vi "Untitled 1.vi"(9 "signal 3":waveform(dbl), 10 "signal 2":waveform(dbl), 11 "signal 1":waveform(dbl)) -> ()   [LabVIEW 2012]
panel:
  out "signal 3":dbl[](array[numeric])
  out "signal 2":dbl[](array[numeric])
  out "t":dbl[](array[numeric])
  out "signal 1":dbl[](array[numeric])
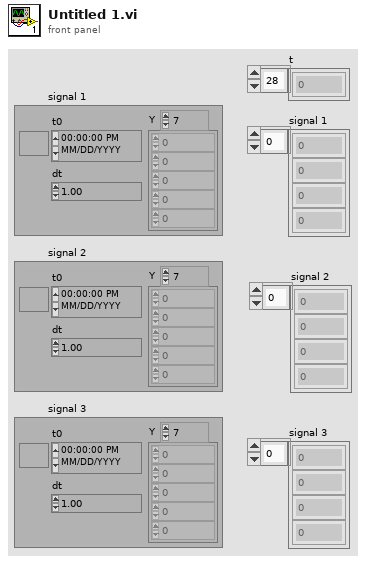
[diagram p1: front panel]
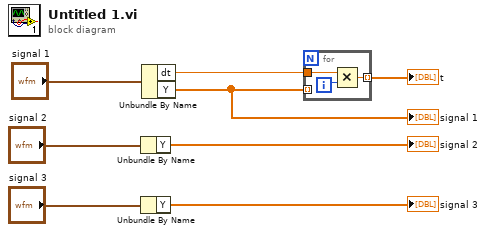
[diagram p0: block diagram]
diagram:
  n1 = Unbundle By Name("signal 2") -> ("Y"=→"signal 2":dbl[])
  n2 = Unbundle By Name("signal 3") -> ("Y"=→"signal 3":dbl[])
  n3 = Unbundle By Name("signal 1") -> ("dt"=w7:dbl, "Y"=w5:dbl[])
  "signal 1" <- w5
  n4 = for {
    tunnel: w7 -> [w11]
    tunnel: w5 -> [_] mode=indexing
    tunnel: [w9] -> w6 mode=indexing
    i -> [w10]
    n5 = Multiply(x=w11, y=w10) -> (x*y=w9:dbl)
  }
  "t" <- w6
